vi "Save Simplified Channel List.vi"(8 "error in (no error)":errorcluster, 11 "VI in":refnum<class "VI.lvclass">) -> (0 "error out":errorcluster, 3 "VI out":refnum<class "VI.lvclass">)   [LabVIEW 2025, in "VI.lvclass"]
doc: "Save a simple csv file that contains the channel order for the debug DMA channel."
uses:
  VI.lvclass
  VI.lvclass/VI.ctl
  Module Loop/Read Modules.vi
  Module/Module/Read Signal List.vi
  Signal/Signal/Read IO Name.vi
  Signal/Signal/Read Signal Name.vi
  Module/Module/Module.lvclass
  Signal/Signal/Signal.lvclass
  Module Loop/Module Loop.lvclass
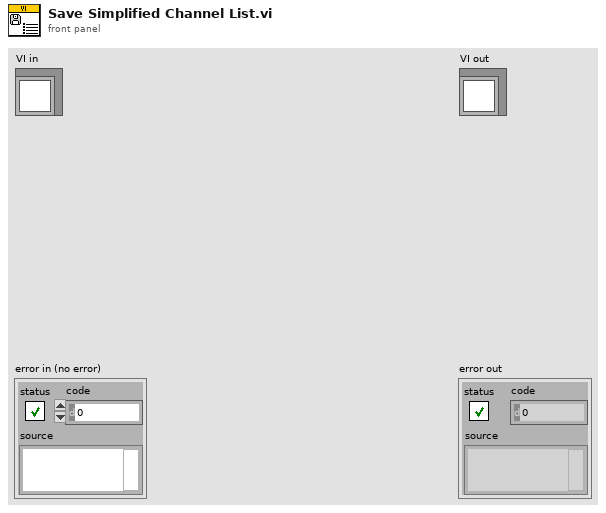
[diagram p1: front panel]
types:
  T1 = enum16{"open", "replace", "create", "open or create", "replace or create", "replace or create with confirmation"}
  T2 = cluster{"IO Name":string, "Signal Name":string}[]
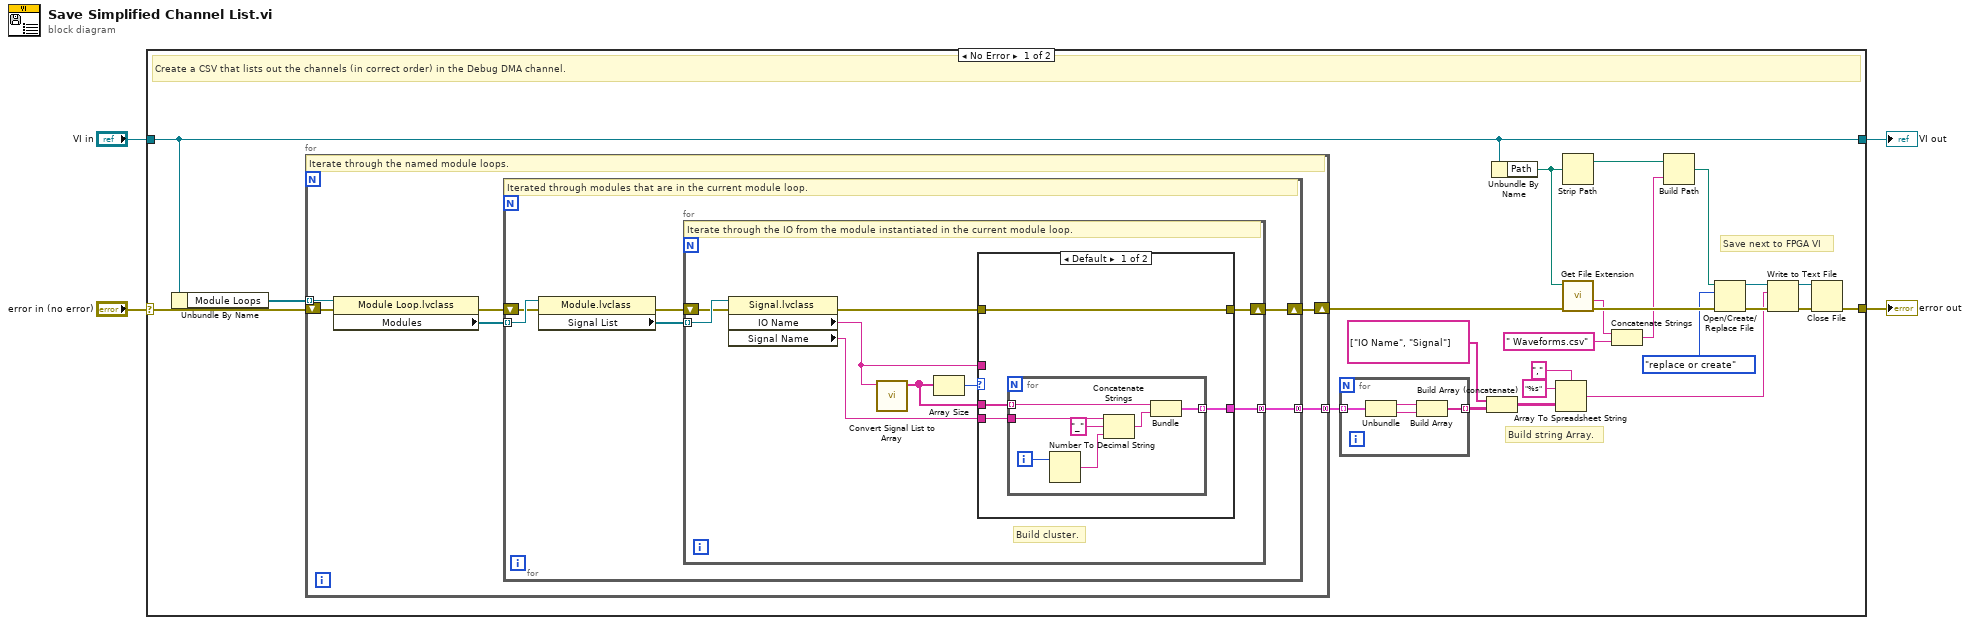
[diagram p0: block diagram]
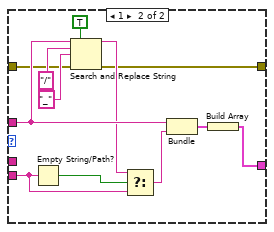
[diagram p2: hidden frame]
diagram:
  n1 = case shown="No Error" "error in (no error)" {
    selector: "error in (no error)" -> [w22 w78]
    tunnel: [w7 w78] -> w3
    tunnel: [w21 w77] -> w1
    tunnel: "VI in" -> [w21 w77]
    frame No Error {
      # "Save next to FPGA VI"
      # "Build string Array."
      # "Create a CSV that lists out the channels (in correct order) in the Debug DMA channel."
      n2 = Unbundle By Name(w21) -> ("Module Loops"=w28:refnum<class "Module Loop.lvclass">[])
      n3 = for {
        tunnel: w28 -> [w38] mode=indexing
        shift-right: [w34] -> w20
        shift-left: w22 -> [w36]
        tunnel: [w33] -> w27 mode=concatenating
        # "Iterate through the named module loops."
        n4 = property class="Module Loop.lvclass"(reference=w38, error in=w36) -> (error out=w35:errorcluster, "Modules"=w37:refnum<class "Module.lvclass">[])  [unwired: 1 out]
        n5 = for {
          tunnel: w37 -> [w44] mode=indexing
          tunnel: [w42] -> w33 mode=concatenating
          shift-right: [w39] -> w34
          shift-left: w35 -> [w41]
          # "Iterated through modules that are in the current module loop."
          n6 = property class="Module.lvclass"(reference=w44, error in=w41) -> (error out=w40:errorcluster, "Signal List"=w43:refnum<class "Signal.lvclass">[])  [unwired: 1 out]
          n7 = for {
            tunnel: w43 -> [w53] mode=indexing
            tunnel: [w49] -> w42 mode=concatenating
            shift-right: [w45] -> w39
            shift-left: w40 -> [w47]
            # "Build cluster."
            # "Iterate through the IO from the module instantiated in the current module loop."
            n8 = property class="Signal.lvclass"(reference=w53, error in=w47) -> (error out=w46:errorcluster, "IO Name"=w51:string, "Signal Name"=w50:string)  [unwired: 1 out]
            n9 = call "Convert Signal List to Array.vi"("Signal List"=w51) -> ("Signal List"=w48:string[])  [unwired: 10 in]
            n10 = Array Size(array=w48) -> (size(s)=w52:i32)
            n11 = case shown="Default" w52 {
              tunnel: w51 -> [_ w73]
              tunnel: w50 -> [w57 w68]
              tunnel: [w55 w75] -> w49
              tunnel: w48 -> [w56 _]
              tunnel: w46 -> [w54 w67]
              tunnel: [w54 w66] -> w45
              frame Default {
                n12 = for {
                  tunnel: w57 -> [w63]
                  tunnel: w56 -> [w59] mode=indexing
                  tunnel: [w58] -> w55 mode=indexing
                  i -> [w64]
                  n13 = Number To Decimal String(number=w64) -> (decimal integer string=w61:string)  [unwired: 1 in]
                  n14 = Concatenate Strings(w63, "_" ("string"), w61) -> (w60:string)
                  n15 = Bundle("trimmed string"=w59, w60) -> (w58:cluster{"trimmed string":string, string})  [unwired: 1 in]
                }
              }
              frame 1 {
                n16 = Empty String/Path?(string/path=w68) -> (empty?=w74:bool)
                n17 = Search and Replace String(replace all?=TRUE ("replace all? (F)"), input string=w73, search string="/", replace string="_" ("replace string (\"\")"), error in=w67) -> (result string=w69:string, error out=w66:errorcluster)  [unwired: 3 in, 2 out]
                n18 = Select(t=w69, s=w74, f=w68) -> (s? t:f=w65:string)
                n19 = Bundle("IO Name"=w73, "Signal Name"=w65) -> (w76:cluster{"IO Name":string, "Signal Name":string})  [unwired: 1 in]
                n20 = Build Array(w76) -> (w75:T2)
              }
            }
          }
        }
      }
      n21 = for {
        tunnel: w27 -> [w32] mode=indexing
        tunnel: [w29] -> w25 mode=indexing
        n22 = Unbundle(w32) -> ("IO Name"=w31:string, "Signal Name"=w30:string)
        n23 = Build Array(w31, w30) -> (w29:string[])
      }
      n24 = Build Array (concatenate)(string[] ["IO Name", "Signal"], w25) -> (w23:string[][])
      n25 = Unbundle By Name(w21) -> ("Path"=w16:path)
      n26 = Array To Spreadsheet String(delimiter (Tab)=",", array=w23, 3:"%s" ("format string")) -> (spreadsheet string=w11:string)
      n27 = Strip Path(path=w16) -> (stripped path=w15:path)  [unwired: 1 out]
      n28 = call <vilib>:"Get File Extension.vi"("error in (no error)"=w20, "file"=w16) -> ("error out"=w19:errorcluster, "filename without extension"=w18:string)  [unwired: 5 in, 3 out]
      n29 = Concatenate Strings(w18, " Waveforms.csv" ("string")) -> (w14:string)
      n30 = Build Path(base path=w15, name or relative path=w14) -> (appended path=w13:path)
      n31 = Open/Create/Replace File(file path (use dialog)=w13, error in=w19, operation (0:open)=T1."replace or create") -> (refnum out=w10:refnum<file>, error out=w12:errorcluster)  [unwired: 3 in, 1 out]
      n32 = Write to Text File(file (use dialog)=w10, text=w11, error in=w12) -> (refnum out=w8:refnum<file>, error out=w9:errorcluster)  [unwired: 1 in, 1 out]
      n33 = Close File(refnum=w8, error in=w9) -> (error out=w7:errorcluster)  [unwired: 1 out]
    }
    frame Error {
    }
  }
  "error out" <- w3
  "VI out" <- w1
